vi "FTW-Actor-OpeningHandshake.vi"(0 "FTW Actor Instance Type":refnum<class "FTW-Actor-Instance.lvclass">, 5 "Initialization Job Sequence":string, 7 "Actor Instance Configuration":string, 11 "error in":errorcluster) -> (4 "FTW Actor Instance":refnum<class "FTW-Actor-Instance.lvclass">, 6 "Incoming Request":refnum<event-registration>, 15 "error out":errorcluster)   [LabVIEW 2014, in "FTW-Actor-Instance.lvclass"]
uses:
  FTW-Actor-Instance.lvclass
  json/FTW-JSON-Deserialize/FTW-JSON-Deserialize.xnode
  json/core/FTW-JSON-Core-GetFlattenedValue.vi
  reflection/FTW-Reflection-Type.vi
  json/FTW-JSON-Destroy.vi
  json/core/FTW-JSON-Core-Structure.ctl
panel:
  # "Inputs"
  # "Outputs"
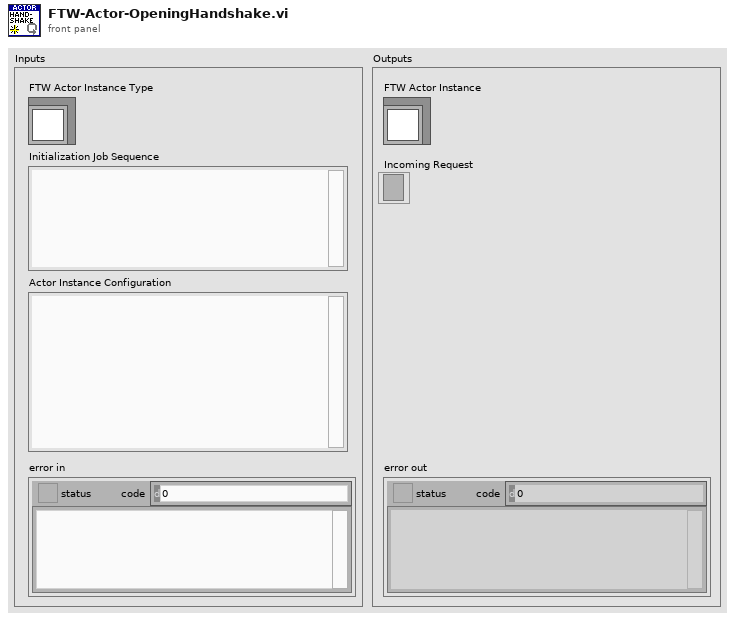
[diagram p1: front panel]
types:
  T1 = cluster{"Identity":string, "InboxAddress":string, "InboxConfiguration":string, "SupervisorAddress":string, "LauncherAddress":string, "DebugEnableInboxLogging":bool, "DebugEnableJobLogging":bool, "LaunchTimeout":i32}
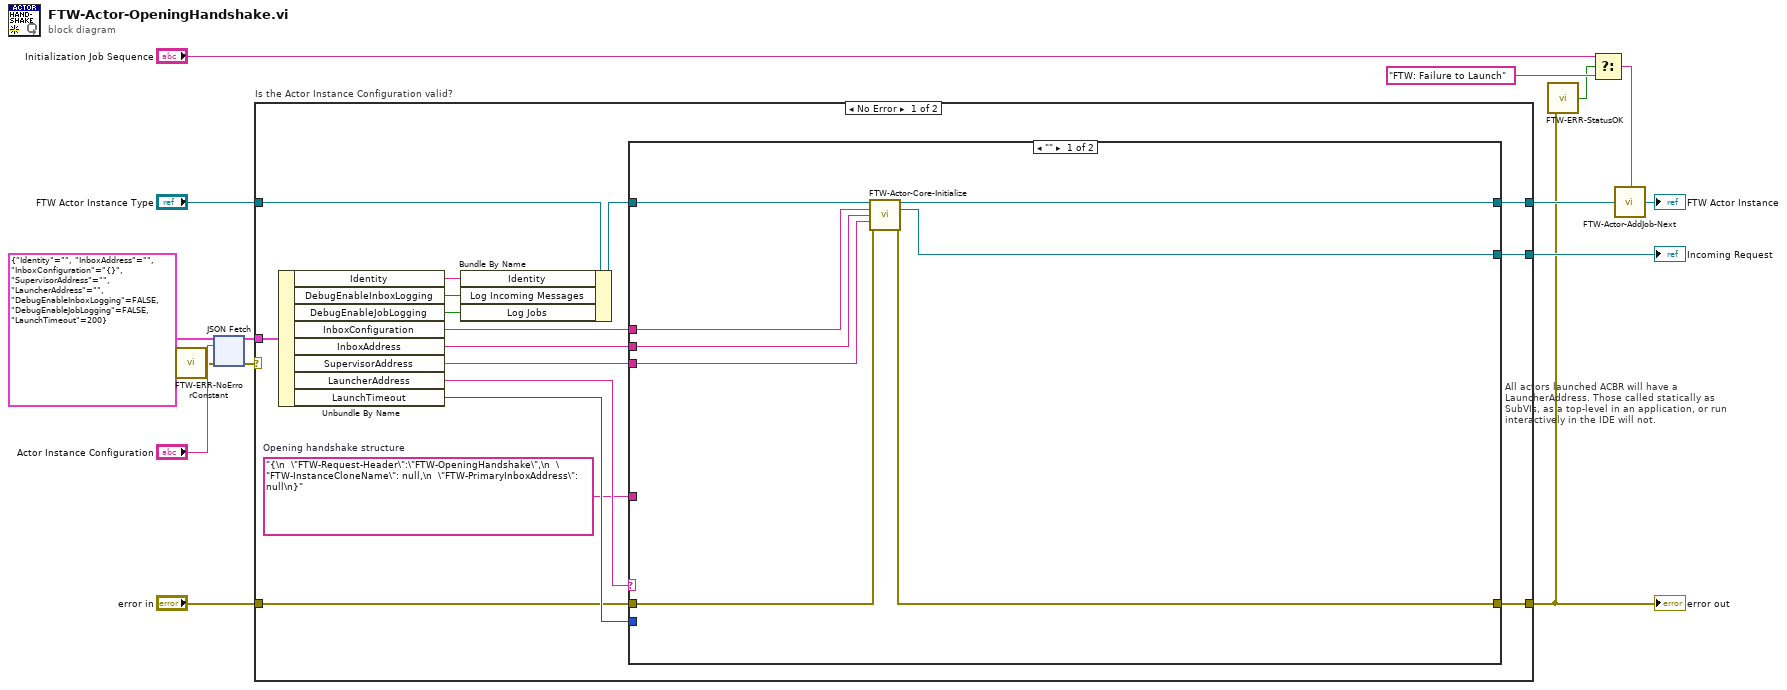
[diagram p0: block diagram]
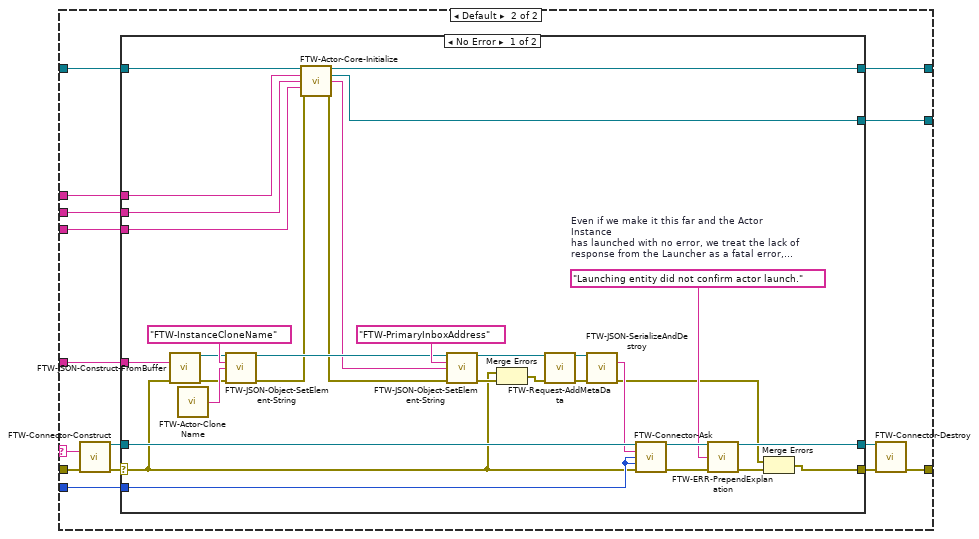
[diagram p2: hidden frame]
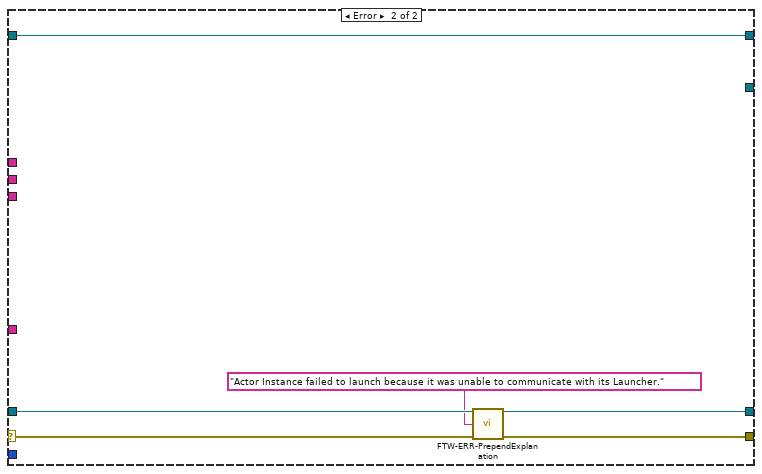
[diagram p3: hidden frame]
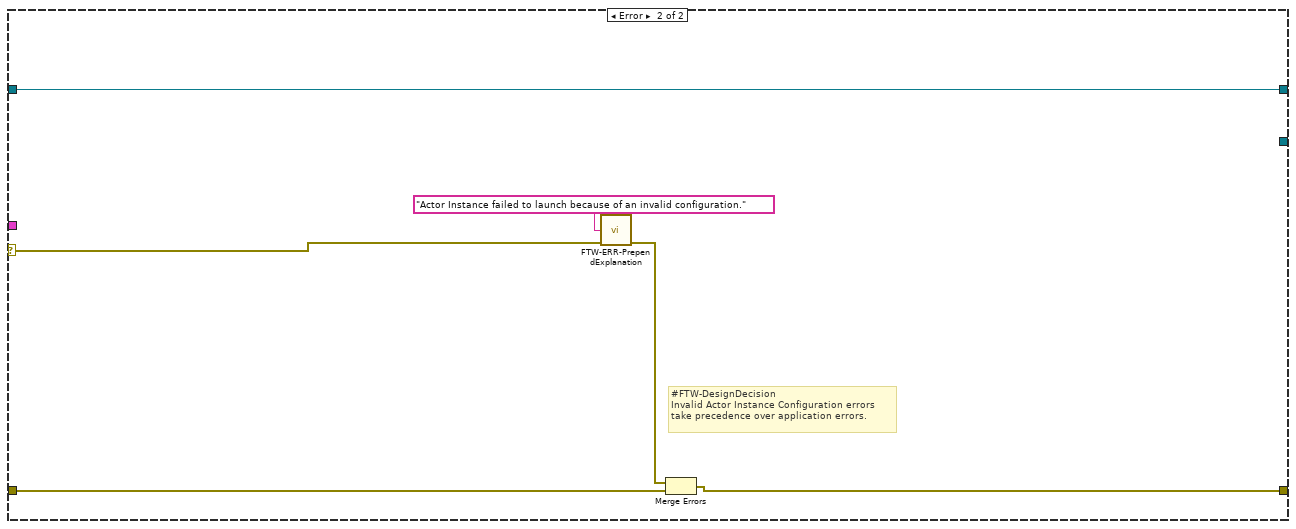
[diagram p4: hidden frame]
diagram:
  n1 = call "FTW-ERR-NoErrorConstant.vi"() -> ("no error"=w10:errorcluster)
  n2 = xnode "JSON Fetch"("Type and Defaults"=T1 {"Identity"="", "InboxAddress"="", "InboxConfiguration"="{}", "SupervisorAddress"="", "LauncherAddress"="", "DebugEnableInboxLogging"=FALSE, "DebugEnableJobLogging"=FALSE, "LaunchTimeout"=200}, "JSON String"="Actor Instance Configuration", "error in"=w10) -> ("Values"=w11:T1, "error out"=w9:errorcluster)  [unwired: 1 in]
  n3 = case "Is the Actor Instance Configuration valid?" shown="No Error" w9 {
    selector: w9 -> [_ w93]
    tunnel: "FTW Actor Instance Type" -> [w23 w96]
    tunnel: [w26 w94] -> w2
    tunnel: [w31 _] -> w14
    tunnel: [w30 w96] -> w7
    tunnel: w11 -> [w29 _]
    tunnel: "error in" -> [w25 w95]
    frame No Error {
      w17 = "{\n  \"FTW-Request-Header\":\"FTW-OpeningHandshake\",\n  \"FTW-InstanceCloneName\": null,\n  \"FTW-PrimaryInboxAddress\": null\n}"  # Opening handshake structure
      n4 = Unbundle By Name(w29) -> ("Identity"=w21:string, "DebugEnableInboxLogging"=w20:bool, "DebugEnableJobLogging"=w19:bool, "InboxConfiguration"=w18:string, "InboxAddress"=w28:string, "SupervisorAddress"=w16:string, "LauncherAddress"=w24:string, "LaunchTimeout"=w27:i32)
      n5 = Bundle By Name(cluster=w23, "Identity"=w21, "Log Incoming Messages"=w20, "Log Jobs"=w19) -> (w22:refnum<class "FTW-Actor-Instance.lvclass">)
      n6 = case "All actors launched ACBR will have a LauncherAddress. Those called statically as SubVIs, as a top-level in an application, or run interactively in the IDE will not." shown="\"\"" w24 {
        selector: w24 -> [_ w42]
        tunnel: w22 -> [w39 w54]
        tunnel: [w33 w53] -> w31
        tunnel: [w38 w52] -> w30
        tunnel: w28 -> [w36 w51]
        tunnel: w27 -> [_ w50]
        tunnel: [w34 w45] -> w26
        tunnel: w25 -> [w35 w44]
        tunnel: w17 -> [_ w43]
        tunnel: w18 -> [w37 w41]
        tunnel: w16 -> [w32 w40]
        frame "" {
          n7 = call "FTW-Actor-Core-Initialize.vi"("FTW Actor Instance"=w39, "Inbox Configuration"=w37, "Primary Inbox Address"=w36, "Supervisor Address"=w32, "error in"=w35) -> ("FTW Actor Instance out"=w38:refnum<class "FTW-Actor-Instance.lvclass">, "Incoming Request"=w33:refnum<event-registration>, "error out"=w34:errorcluster)  [unwired: 7 in, 1 out]
        }
        frame Default {
          n8 = call "FTW-Connector-Construct.vi"("Remote Inbox Address"=w42, "error in"=w44) -> ("FTW Actor Connector"=w49:refnum<data-value>, "error out"=w48:errorcluster)  [unwired: 12 in]
          n9 = case shown="No Error" w48 {
            selector: w48 -> [w70 w88]
            tunnel: w54 -> [w63 w89]
            tunnel: [w64 w87] -> w46
            tunnel: [w61 _] -> w53
            tunnel: [w57 w89] -> w52
            tunnel: w51 -> [w56 _]
            tunnel: w50 -> [w84 _]
            tunnel: w49 -> [w83 w90]
            tunnel: [w82 w90] -> w47
            tunnel: w43 -> [w68 _]
            tunnel: w41 -> [w62 _]
            tunnel: w40 -> [w55 _]
            frame No Error {
              w69 = "Launching entity did not confirm actor launch."  # Even if we make it this far and the Actor Instance has launched with no error, we treat the lack of response from the Launcher as a fatal error, such that this Actor Instance does not exist as a renegade.
              n10 = call "FTW-JSON-Construct-FromBuffer.vi"("JSON String (UTF-8)"=w68, "error in"=w70) -> ("JSON Object"=w76:refnum<data-value>, "error out"=w75:errorcluster)  [unwired: 12 in]
              n11 = call "FTW-Actor-CloneName.vi"() -> ("Clone Name"=w85:string)  [unwired: 1 in]
              n12 = call "FTW-JSON-Object-SetElement-String.vi"("JSON Object"=w76, "Key"="FTW-InstanceCloneName", "Value"=w85, "error in"=w75) -> ("JSON Object out"=w74:refnum<data-value>, "error out"=w59:errorcluster)  [unwired: 10 in]
              n13 = call "FTW-Actor-Core-Initialize.vi"("FTW Actor Instance"=w63, "Inbox Configuration"=w62, "Primary Inbox Address"=w56, "Supervisor Address"=w55, "error in"=w59) -> ("FTW Actor Instance out"=w57:refnum<class "FTW-Actor-Instance.lvclass">, "Incoming Request"=w61:refnum<event-registration>, "Resolved Primary Inbox Address"=w60:string, "error out"=w58:errorcluster)  [unwired: 7 in]
              n14 = call "FTW-JSON-Object-SetElement-String.vi"("JSON Object"=w74, "Key"="FTW-PrimaryInboxAddress", "Value"=w60, "error in"=w58) -> ("JSON Object out"=w72:refnum<data-value>, "error out"=w71:errorcluster)  [unwired: 10 in]
              n15 = Merge Errors(w70, w71) -> (w79:errorcluster)
              n16 = call "FTW-Request-AddMetaData.vi"("Response"=w72, "error in"=w79) -> ("Response out"=w81:refnum<data-value>, "error out"=w73:errorcluster)  [unwired: 12 in]
              n17 = call "FTW-JSON-SerializeAndDestroy.vi"("JSON Object"=w81, "error in"=w73) -> ("JSON String (UTF-8)"=w80:string, "error out"=w67:errorcluster)  [unwired: 12 in]
              n18 = call "FTW-Connector-Ask.vi"("FTW Actor Connector"=w83, "Request"=w80, "Receive Timeout"=w84, "Send Timeout"=w84, "error in"=w70) -> ("FTW Actor Connector out"=w82:refnum<data-value>, "error out"=w66:errorcluster)  [unwired: 7 in, 2 out]
              n19 = call "FTW-ERR-PrependExplanation.vi"("Exception Information"=w69, "error in"=w66) -> ("error out"=w65:errorcluster)  [unwired: 13 in]
              n20 = Merge Errors(w67, w65) -> (w64:errorcluster)
            }
            frame Error {
              n21 = call "FTW-ERR-PrependExplanation.vi"("Exception Information"="Actor Instance failed to launch because it was unable to communicate with its Launcher." ("Error Message"), "error in"=w88) -> ("error out"=w87:errorcluster)  [unwired: 13 in]
            }
          }
          n22 = call "FTW-Connector-Destroy.vi"("FTW Connector"=w47, "error in"=w46) -> ("error out"=w45:errorcluster)  [unwired: 13 in]
        }
      }
    }
    frame Error {
      # "#FTW-DesignDecision\nInvalid Actor Instance Configuration errors\ntake precedence over application errors."
      n23 = call "FTW-ERR-PrependExplanation.vi"("Exception Information"="Actor Instance failed to launch because of an invalid configuration." ("Error Message"), "error in"=w93) -> ("error out"=w92:errorcluster)  [unwired: 13 in]
      n24 = Merge Errors(w92, w95) -> (w94:errorcluster)
    }
  }
  "error out" <- w2
  "Incoming Request" <- w14
  n25 = call "FTW-ERR-StatusOK.vi"("error to check"=w2) -> ("Status OK?"=w3:bool)
  n26 = Select(t="Initialization Job Sequence", s=w3, f="FTW: Failure to Launch") -> (s? t:f=w1:string)
  n27 = call "FTW-Actor-AddJob-Next.vi"("Add Next in Job Queue"=w1, "FTW Actor Instance"=w7) -> ("FTW Actor Instance out"=→"FTW Actor Instance":refnum<class "FTW-Actor-Instance.lvclass">)  [unwired: 2 in]
